vi "TransportWrapper.vi"(4 "ReplyLength":i32=2147483647, 6 "ReplyFirstByte":T1=224 items=["-1"=224, "DIGITAL_IO_MESSAGE"=144, "REPORT_ANALOG_PIN"=192, "REPORT_DIGITAL_PORT"=208, "START_SYSEX"=240, "END_SYSEX"=247, "SET_PIN_MODE"=244, "SET_DIGITAL_PIN_VALUE"=245, "PROTOCOL_VERSION"=249, "SYSTEM_RESET"=255, "SYSEX.EXTENDED_ID"=0, "SYSEX.RESERVED_USER_COMMANDs"=1, "SYSEX.ANALOG_MAPPING_QUERY"=105, "SYSEX.ANALOG_MAPPING_RESPONSE"=106, "SYSEX.CAPABILITY_QUERY"=107, "SYSEX.CAPABILITY_RESPONSE"=108, "SYSEX.PIN_STATE_QUERY"=109, "SYSEX.PIN_STATE_RESPONSE"=110, "SYSEX.REPORT_FIRMWARE"=121, "SYSEX.EXTENDED_ANALOG"=111, "SYSEX.STRING_DATA"=113, "SYSEX.REALTIME"=127, "SYSEX.NON_REALTIME"=126, "SYSEX.SAMPLING_INTERVAL"=122, "FEATURES.SYSEX.I2C_READ_WRITE"=118, "FEATURES.SYSEX.I2C_REPLY"=119, "FEATURES.SYSEX.I2C_CONFIG"=120], 8 "error in":errorcluster, 10 "Message In":u8[](array[numeric]) format="%x", 11 "Refnum In":refnum<vi>) -> (0 "error out":errorcluster, 2 "Message Out":u8[](array[numeric]) format="%x", 3 "Refnum Out":refnum<vi>)   [LabVIEW 2020]
doc: "Performs some preprocessing before using the selected transport metod to send and / or receive data. It will also perform some post processing after receiving the data.\nProcessing consist of light packaging / formatting"
uses:
  Controls/FirmataProtocolConstants.ctl
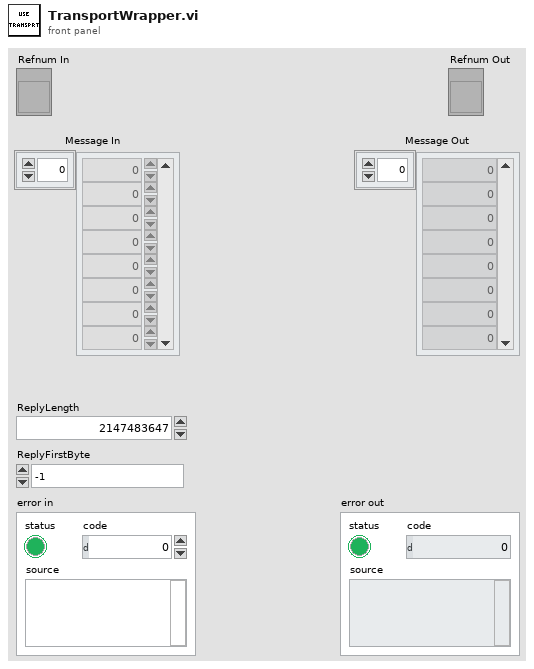
[diagram p1: front panel]
types:
  T1 = typedef "FirmataProtocolConstants.ctl" = u16
  T2 = typedef "Parameters.ctl" = cluster{"Transport Parameters":T3, "Board Capabilities":map{i32, T5}}
  T3 = typedef "TransportParameters.ctl" = cluster{"Serial Communication":cluster{"Comport":refnum<visa-resource-name>, "No Response Timeout Ms":u32, "Response Complete Timeout Ms":u32, "Max Rx Length":u32, "Baud Rate":u32}, "Selected Transport":T4, "Initializer File Path":path, "Cleaner File Path":path, "Transporter File Path":path}
  T4 = typedef "SupportedTransports.ctl" = enum16{"Serial Communication Port"}
  T5 = typedef "FirmataPinCapabilitiesAndAnalogMapping.ctl" = cluster{"Supported Modes":T6[], "Analog Channel":u8, "Pin Name":string}
  T6 = typedef "FirmataPinCapability.ctl" = cluster{"PinMode":T7, "Resolution":u8}
  T7 = typedef "FirmataPinModes.ctl" = enum16{"DigitalInput", "DigitalOutput", "AnalogInput", "PWM", "Servo", "Shift", "I2C", "OneWire", "Stepper", "Encoder", "Serial", "InputPullup", "Extended.SPI", "Extended.Sonar", "Extended.Tone", "Extended.DHT"}
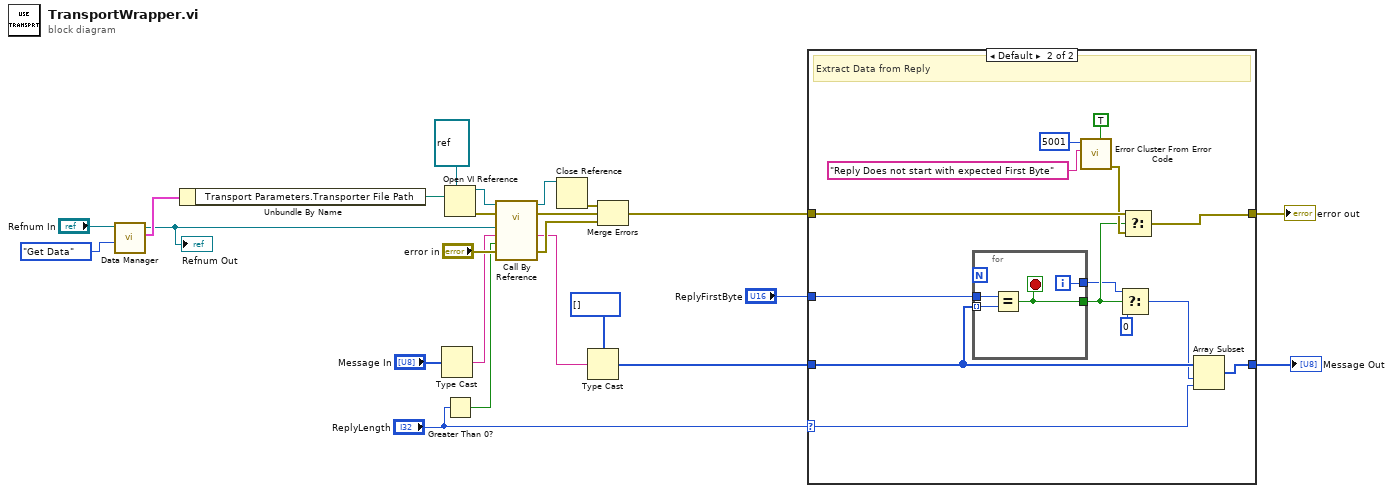
[diagram p0: block diagram]
diagram:
  n1 = call "Data Manager.vi"("Mode"=enum16{"Store Data", "Get Data", "Cleanup"}."Get Data", "Refnum In"="Refnum In") -> ("Data Out"=w14:T2, "Refnum Out"=w3:refnum<vi>)  [unwired: 7 in, 1 out]
  "Refnum Out" <- w3
  n2 = Unbundle By Name(w14) -> ("Transport Parameters.Transporter File Path"=w16:path)
  n3 = Type Cast(x="Message In") -> (*(type *) &x=w11:string)  [unwired: 1 in]
  n4 = Open VI Reference(type specifier VI Refnum (for type only)=refnum<vi> refnum, vi path=w16) -> (vi reference=w22:refnum<vi>, error out=w23:errorcluster)  [unwired: 4 in]
  n5 = Greater Than 0?(x="ReplyLength") -> (x > 0?=w1:bool)
  n6 = call-by-ref "?"(reference=w22, error in=w23, "error in"="error in", "Wait For Response?"=w1, "Message In"=w11, "Refnum In"=w3) -> (reference out=w21:refnum<vi>, error out=w19:errorcluster, 0:"error out"=w17:errorcluster, "Message Out"=w10:string)  [unwired: 5 in, 1 out]
  n7 = Close Reference(reference=w21) -> (error out=w18:errorcluster)  [unwired: 1 in]
  n8 = Type Cast(type=u8[] [] ("GetFirmwareMessage"), x=w10) -> (*(type *) &x=w7:u8[])
  n9 = Merge Errors(w18, w19, w17) -> (w5:errorcluster)
  n10 = case shown="Default" "ReplyLength" {
    selector: "ReplyLength" -> [_ w27]
    tunnel: [w26 w40] -> w8
    tunnel: w7 -> [w26 w39]
    tunnel: "ReplyFirstByte" -> [_ w38]
    tunnel: w5 -> [w25 w37]
    tunnel: [w25 w32] -> w4
    frame 0 {
      # "No Reply Expected"
    }
    frame Default {
      # "Extract Data from Reply"
      n11 = for {
        tunnel: w38 -> [w44]
        tunnel: w39 -> [w43] mode=indexing
        tunnel: [w42] -> w31
        tunnel: [w41] -> w30
        i -> [w41]
        stop <- w42 stop-if-true
        n12 = Equal?(x=w44, y=w43) -> (x = y?=w42:bool)
      }
      n13 = call <vilib>:"Error Cluster From Error Code.vi"("is warning? (False)"=TRUE, "error message (\"\")"="Reply Does not start with expected First Byte" ("error message (\"\")"), "error code (0)"=5001) -> ("error out"=w36:errorcluster)  [unwired: 6 in]
      n14 = Select(t=w30, s=w31, f=0) -> (s? t:f=w28:i32)
      n15 = Select(t=w37, s=w31, f=w36) -> (s? t:f=w32:errorcluster)
      n16 = Array Subset(array=w39, index=w28, length=w27) -> (w40:u8[])
    }
  }
  "error out" <- w4
  "Message Out" <- w8
